vi "disconnect.vi"(8 "error in (no error)":errorcluster, 11 "MotorController in":refnum<class "MotorController.lvclass">) -> (0 "error out":errorcluster, 3 "MotorController out":refnum<class "MotorController.lvclass">)   [LabVIEW 2019, in "MotorController.lvclass"]
uses:
  MotorController.lvclass
  MotorController.lvclass/MotorController.ctl
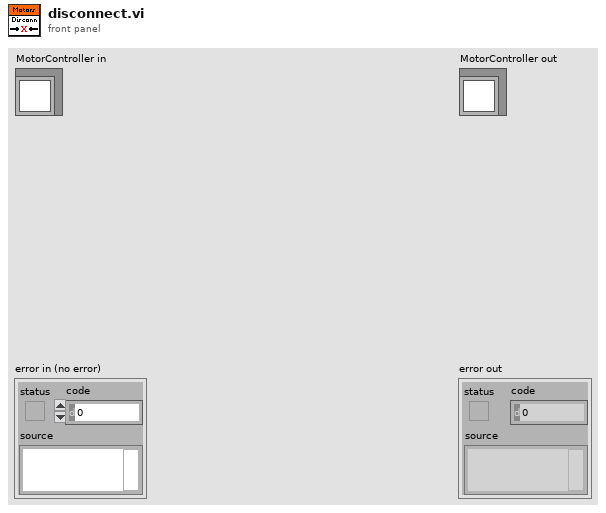
[diagram p1: front panel]
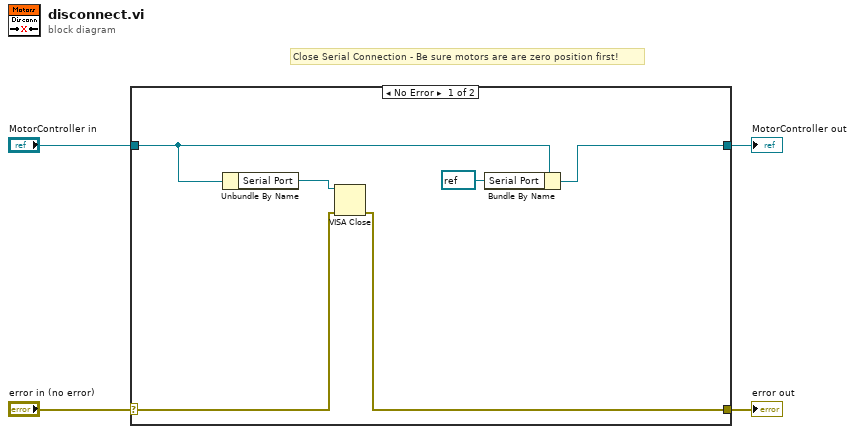
[diagram p0: block diagram]
diagram:
  # "Close Serial Connection - Be sure motors are are zero position first!"
  n1 = case shown="No Error" "error in (no error)" {
    selector: "error in (no error)" -> [w8 w12]
    tunnel: [w7 w12] -> w3
    tunnel: [w5 w11] -> w1
    tunnel: "MotorController in" -> [w10 w11]
    frame No Error {
      n2 = Unbundle By Name(w10) -> ("Serial Port"=w9:refnum<visa-resource-name>)
      n3 = VISA Close(VISA resource name=w9, error in (no error)=w8) -> (error out=w7:errorcluster)
      n4 = Bundle By Name(cluster=w10, "Serial Port"=refnum<visa-resource-name> refnum) -> (w5:refnum<class "MotorController.lvclass">)
    }
    frame Error {
    }
  }
  "error out" <- w3
  "MotorController out" <- w1
